vi "Day 22 - Monkey Map.vi"() -> ()   [LabVIEW 2020, in "AoC 2022.lvlib"]
uses:
  AoC 2022.lvlib
  private/Map Tile.ctl
  private/Map Action Step.ctl
  private/Map Action.ctl
  private/Map Direction.ctl
  Day 15 - Beacon Exclusion Zone/private/Location.ctl
panel:
  out "Steps":T1[](array[typedef])
  out "Map Travel":T4[][][](array[typedef]) items=["Empty", "Portal", "Open", "Wall", ">", "<", ">-^", ">-v", "^-<", "v-<"]
  in  "Puzzle Input":string="        ...#\n        .#..\n        #...\n        ....\n...#.......#\n........#...\n..#....#....\n..........#.\n        ...#....\n        .....#..\n        .#......\n        ......#.\n\n10R5L5R10L4R5L5"
  out "Puzzle Part-2 Answer":string
  out "Puzzle Answer":string
  # "Action"
  # "Direction"
  # "Movement"
  # "Press Ctrl+M & Enter the Puzzle Input and run the VI"
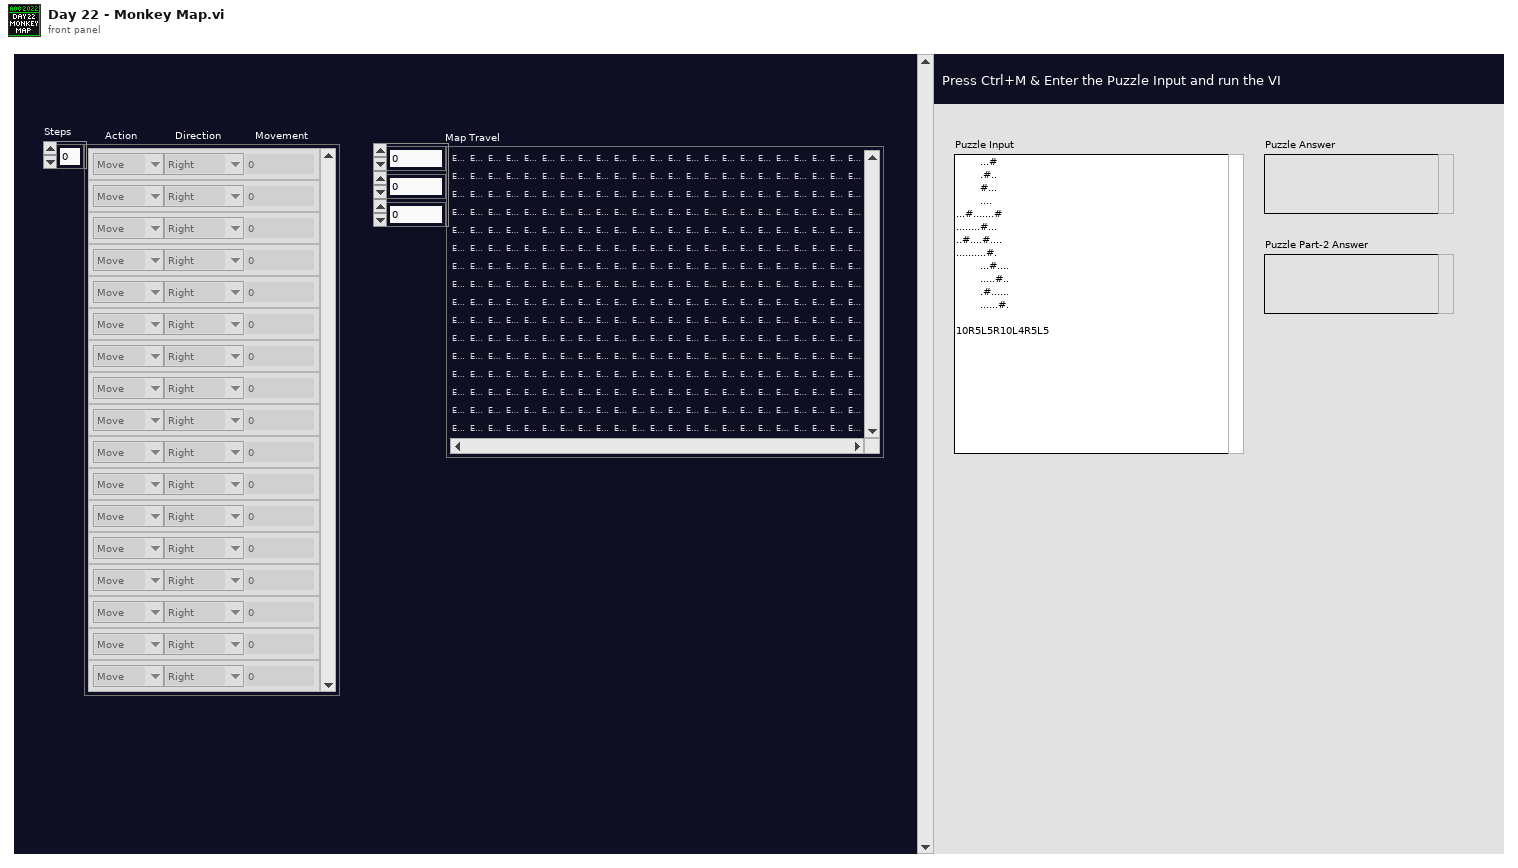
[diagram p1: front panel]
types:
  T1 = typedef "AoC 2022.lvlib/Map Action Step.ctl" = cluster{"Action":T2, "Direction":T3, "Movement":i32}
  T2 = typedef "AoC 2022.lvlib/Map Action.ctl" = enum16{"Move", "Turn"}
  T3 = typedef "AoC 2022.lvlib/Map Direction.ctl" = enum16{"Facing", "Right", "Left", "Up", "Down"}
  T4 = typedef "AoC 2022.lvlib/Map Tile.ctl" = u16
  T5 = typedef "AoC 2022.lvlib/Location.ctl" = cluster{"X":i32, "Y":i32}
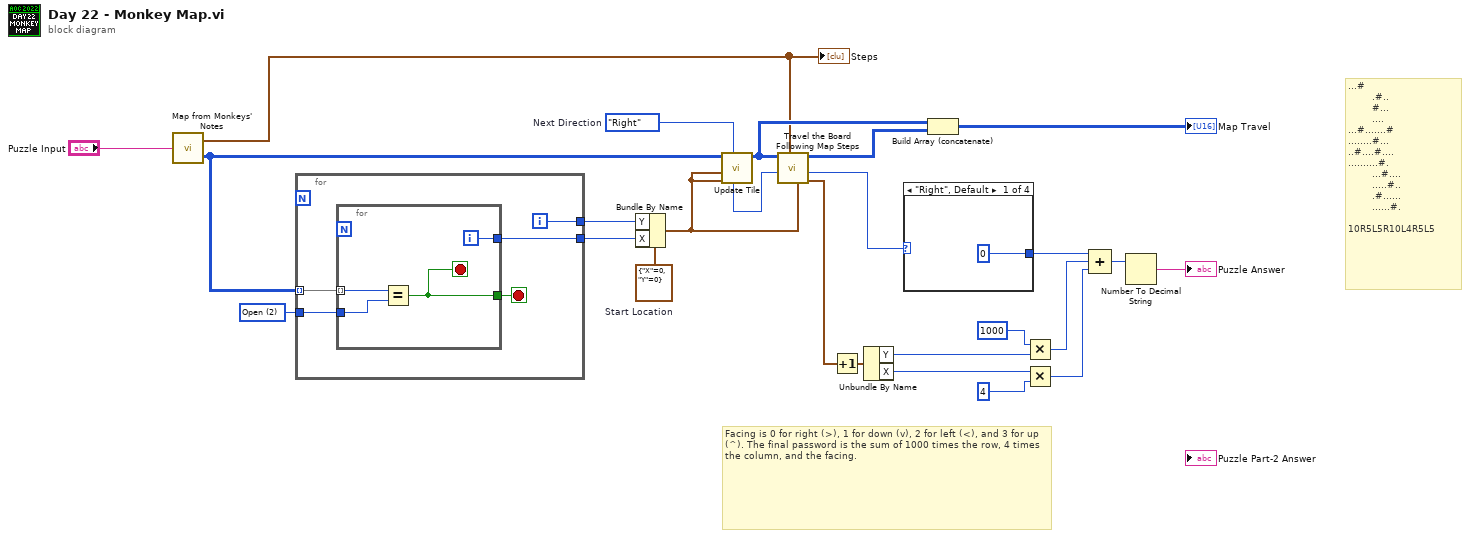
[diagram p0: block diagram]
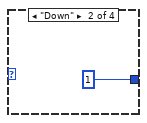
[diagram p2: hidden frame]
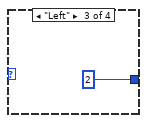
[diagram p3: hidden frame]
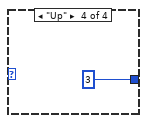
[diagram p4: hidden frame]
diagram:
  w1 = Map_Direction."Right"  # Next Direction
  w21 = T5 {"X"=0, "Y"=0}  # Start Location
  w23 = T4 2 items=["Empty", "Portal", "Open", "Wall", ">", "<", ">-^", ">-v", "^-<", "v-<"]
  # "Facing is 0 for right (>), 1 for down (v), 2 for left (<), and 3 for up (^). The final password is the sum of 1000 times the row, 4 times the column, and the facing."
  # "...#\n        .#..\n        #...\n        ....\n...#.......#\n........#...\n..#....#....\n..........#.\n        ...#....\n        .....#..\n        .#......\n        ......#.\n\n10R5L5R10L4R5L5"
  n1 = call "Map from Monkeys' Notes.vi"("Puzzle Input"="Puzzle Input") -> ("Steps"=w14:T1[], "Board Map"=w22:T4[][])
  "Steps" <- w14
  n2 = for {
    tunnel: w22 -> [w29] mode=indexing
    tunnel: w23 -> [w27]
    tunnel: [w26] -> w20
    tunnel: [w25] -> w19
    i -> [w26]
    stop <- w28 stop-if-true
    n3 = for {
      tunnel: w29 -> [w33] mode=indexing
      tunnel: [w32] -> w28
      tunnel: w27 -> [w31]
      tunnel: [w30] -> w25
      i -> [w30]
      stop <- w32 stop-if-true
      n4 = Equal?(x=w33, y=w31) -> (x = y?=w32:bool)
    }
  }
  n5 = Bundle By Name(cluster=w21, "Y"=w20, "X"=w19) -> (w15:T5)
  n6 = call "Update Tile.vi"("Turn Direction"=w1, "Current Location"=w15, "Next Location"=w15, "Board Map in"=w22) -> ("Board Map out"=w17:T4[][])  [unwired: 4 in, 1 out]
  n7 = call "Travel the Board Following Map Steps.vi"("Start Location"=w15, "Steps"=w14, "Facing Direction in"=w1, "Board Map"=w17) -> ("Last Location"=w13:T5, "Facing Direction out"=w12:T3, "Board Travel"=w18:T4[][][])  [unwired: 3 in]
  n8 = Increment(x=w13) -> (x+1=w2:T5)
  n9 = Unbundle By Name(w2) -> ("Y"=w11:i32, "X"=w9:i32)
  n10 = case shown="\"Right\", Default" w12 {
    tunnel: [0 1 2 3] -> w7
    frame "Right", Default {
    }
    frame "Down" {
    }
    frame "Left" {
    }
    frame "Up" {
    }
  }
  n11 = Build Array (concatenate)(w17, w18) -> (→"Map Travel":T4[][][])
  n12 = Multiply(x=1000, y=w11) -> (x*y=w6:i32)
  n13 = Multiply(x=w9, y=4) -> (x*y=w5:i32)
  n14 = Compound Arithmetic op=ADD(w7, w6, w5) -> (w4:i32)
  n15 = Number To Decimal String(number=w4) -> (decimal integer string=→"Puzzle Answer":string)  [unwired: 1 in]
